vi "IsMoving.vi"(3 "error in (no error)":errorcluster, 5 "StepperController in":refnum<class "StepperController.lvclass">) -> (0 "error out":errorcluster, 1 "IsMoving":bool, 2 "StepperController out":refnum<class "StepperController.lvclass">)   [LabVIEW 2013, in "StepperController.lvclass"]
uses:
  StepperController.lvclass
  StepperController.lvclass/StepperController.ctl
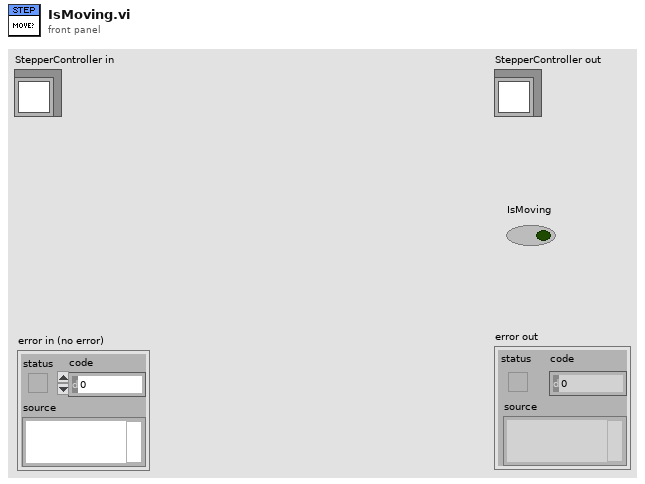
[diagram p1: front panel]
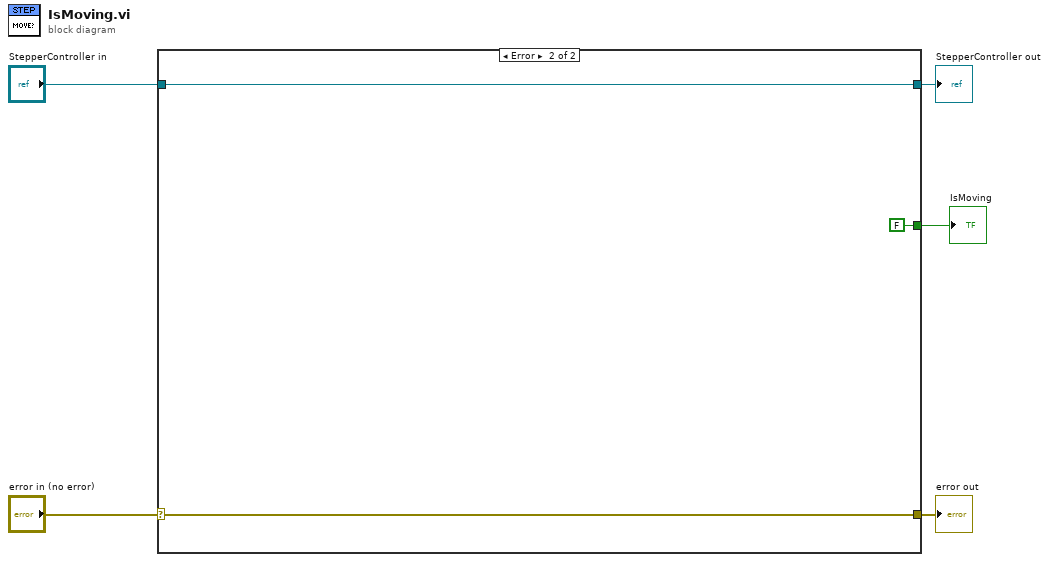
[diagram p0: block diagram]
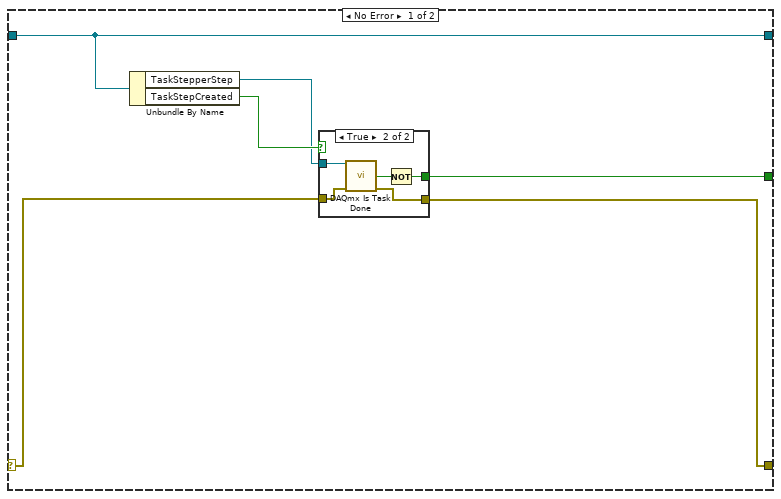
[diagram p2: hidden frame]
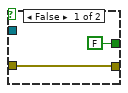
[diagram p3: hidden frame]
diagram:
  n1 = case shown="Error" "error in (no error)" {
    selector: "error in (no error)" -> [w7 w20]
    tunnel: [w6 w20] -> w4
    tunnel: [w10 w21] -> w2
    tunnel: "StepperController in" -> [w10 w21]
    tunnel: [w11 FALSE ("task done?")] -> w1
    frame No Error {
      n2 = Unbundle By Name(w10) -> ("TaskStepperStep"=w8:refnum<k21>, "TaskStepCreated"=w9:bool)
      n3 = case shown="True" w9 {
        tunnel: [FALSE ("task done?") w14] -> w11
        tunnel: w8 -> [_ w18]
        tunnel: w7 -> [w12 w17]
        tunnel: [w12 w16] -> w6
        frame False {
        }
        frame True {
          n4 = call <vilib>:"DAQmx Is Task Done.vi"("task/channels in"=w18, "error in"=w17) -> ("task done?"=w15:bool, "error out"=w16:errorcluster)  [unwired: 11 in, 1 out]
          n5 = Not(x=w15) -> (.not. x?=w14:bool)
        }
      }
    }
    frame Error {
    }
  }
  "error out" <- w4
  "StepperController out" <- w2
  "IsMoving" <- w1
